vi "Periodic Tasks.vi"(8 "error in":errorcluster) -> ()   [LabVIEW 2013]
doc: "This VI runs in parallel to other tasks. It can contain as many user-defined periodic loops as you need. These can carry out PID or other sorts of timed response."
uses:
  <vilib>/Rock Robotics/SystemInterfaces/Utilities/FPGA_UtilitiesLED Source.ctl
  <vilib>/Rock Robotics/SystemInterfaces/Utilities/FPGA_UtilitiesLED State.ctl
  Robot Global Data.vi
  <vilib>/Rock Robotics/WPI/RobotDrive/WPI_RobotDriveArcadeDrive_Standard(NoSaturation).vi
panel:
  out "Rear Motor Run?":bool
  out "Front LEFT Motor Output  2":dbl
  out "Rear RIGHT Motor Output 2":dbl
  out "Front Left Net Closed?":bool
  out "Front Left Net Open?":bool
  out "Rear Right Net Closed?":bool
  out "Rear Right Net Open?":bool
  out "Front LEFT Motor Output":dbl
  out "Rear RIGHT Motor Output":dbl
  out "axis 4":dbl
  out "axis 3 (throttle)":dbl
  out "Ball Motor Output":dbl
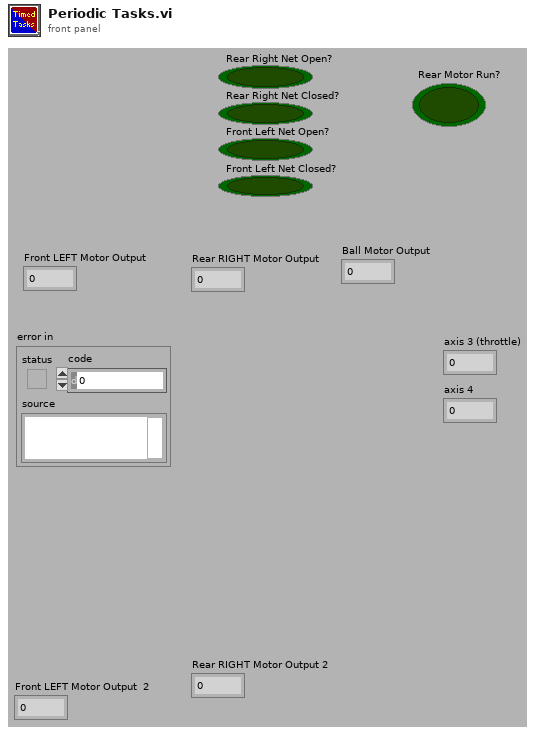
[diagram p1: front panel]
types:
  T1 = typedef "WPI_DigitalInputDevRef.ctl" = cluster{"DevStatus":errorcluster, "DIO Channel":T2, "Digital Module":T3}
  T2 = typedef "FPGA_DIOChannel.ctl" = enum8{"DIO 1", "DIO 2", "DIO 3", "DIO 4", "DIO 5", "DIO 6", "DIO 7", "DIO 8", "DIO 9", "DIO 10", "DIO 11", "DIO 12", "DIO 13", "DIO 14", "Invalid"}
  T3 = typedef "FPGA_TypedefDigitalModule.ctl" = enum16{"Digital Module 1", "Digital Module 2"}
  T4 = typedef "WPI_MotorControlDeviceRef.ctl" = cluster{"DeviceStatus":errorcluster, "Type":enum16{"PWM", "CAN"}, "PWM":cluster{"Digital Module":T3, "PWM Channel":T5, "DeadBand":T6}, "CAN":cluster{"Device Number":u8, "Control Mode":T7, "Semaphore":T8, "Max Vout":dbl}, "Invert":bool, "TransformRef":T9, "InvTransformRef":T9}
  T5 = typedef "FPGA_DIOPWMChannel.ctl" = enum8{"PWM 1", "PWM 2", "PWM 3", "PWM 4", "PWM 5", "PWM 6", "PWM 7", "PWM 8", "PWM 9", "PWM 10", "Invalid"}
  T6 = typedef "WPI_PWMDeadband.ctl" = cluster{"Name":string, "maxPositivePwm":i32, "minPositivePwm":i32, "centerPwm":i32, "maxNegativePwm":i32, "minNegativePwm":i32, "angularRange":u16}
  T7 = typedef "WPI_CANJaguar_ControlMode.ctl" = enum8{"Percent VBus", "Current", "Speed", "Position", "Voltage"}
  T8 = typedef "Semaphore RefNum" = refnum<k1>
  T9 = typedef "WPI_PWMTransform_ConPane.ctl" = refnum<vi>
  T10 = typedef "WPI_JoystickDevRef.ctl" = cluster{"Device":T11}
  T11 = typedef "WPI_JoystickDeviceEnum.ctl" = enum16{"USB 1", "USB 2", "USB 3", "USB 4", "Kinect 1", "Kinect 2"}
  T12 = typedef "WPI_RobotDriveDevRef.ctl" = cluster{"DevStatus":errorcluster, "Motors[]":T4[], "Square Inputs":bool, "Max Output":dbl, "Isochronous":bool}
  T13 = typedef "WPI_GyroDevRef.ctl" = cluster{"DevStatus":errorcluster, "Analog Module":T14, "Analog Channel":T15, "Offset":dbl, "Gain (VoltsPerDegree/Second)":dbl}
  T14 = typedef "FPGA_TypedefAnalogModule.ctl" = enum16{"Analog Module 1", "Analog Module 2"}
  T15 = typedef "FPGA_AIChannel.ctl" = enum8{"AI 1", "AI 2", "AI 3", "AI 4", "AI 5", "AI 6", "AI 7", "AI 8", "Invalid"}
  T16 = typedef "WPI_AnalogChannelDevRef.ctl" = cluster{"DevStatus":errorcluster, "Analog Module":T14, "Analog Channel":T15}
  T17 = typedef "FPGA_UtilitiesLED State.ctl" = enum16{"Off", "On", "Toggle"}
  T18 = typedef "FPGA_UtilitiesLED Source.ctl" = enum16{"User LED", "FPGA LED"}
  T19 = cluster{"axis 1 (x)":dbl, "axis 2 (y)":dbl, "axis 3 (throttle)":dbl, "axis 4":dbl, "axis 5":dbl, "axis 6":dbl}
  T20 = typedef "WPI_JoystickButtonState.ctl" = cluster{"Button 1":bool, "Button 2":bool, "Button 3":bool, "Button 4":bool, "Button 5":bool, "Button 6":bool, "Button 7":bool, "Button 8":bool, "Button 9":bool, "Button 10":bool, "Button 11":bool, "Button 12":bool}
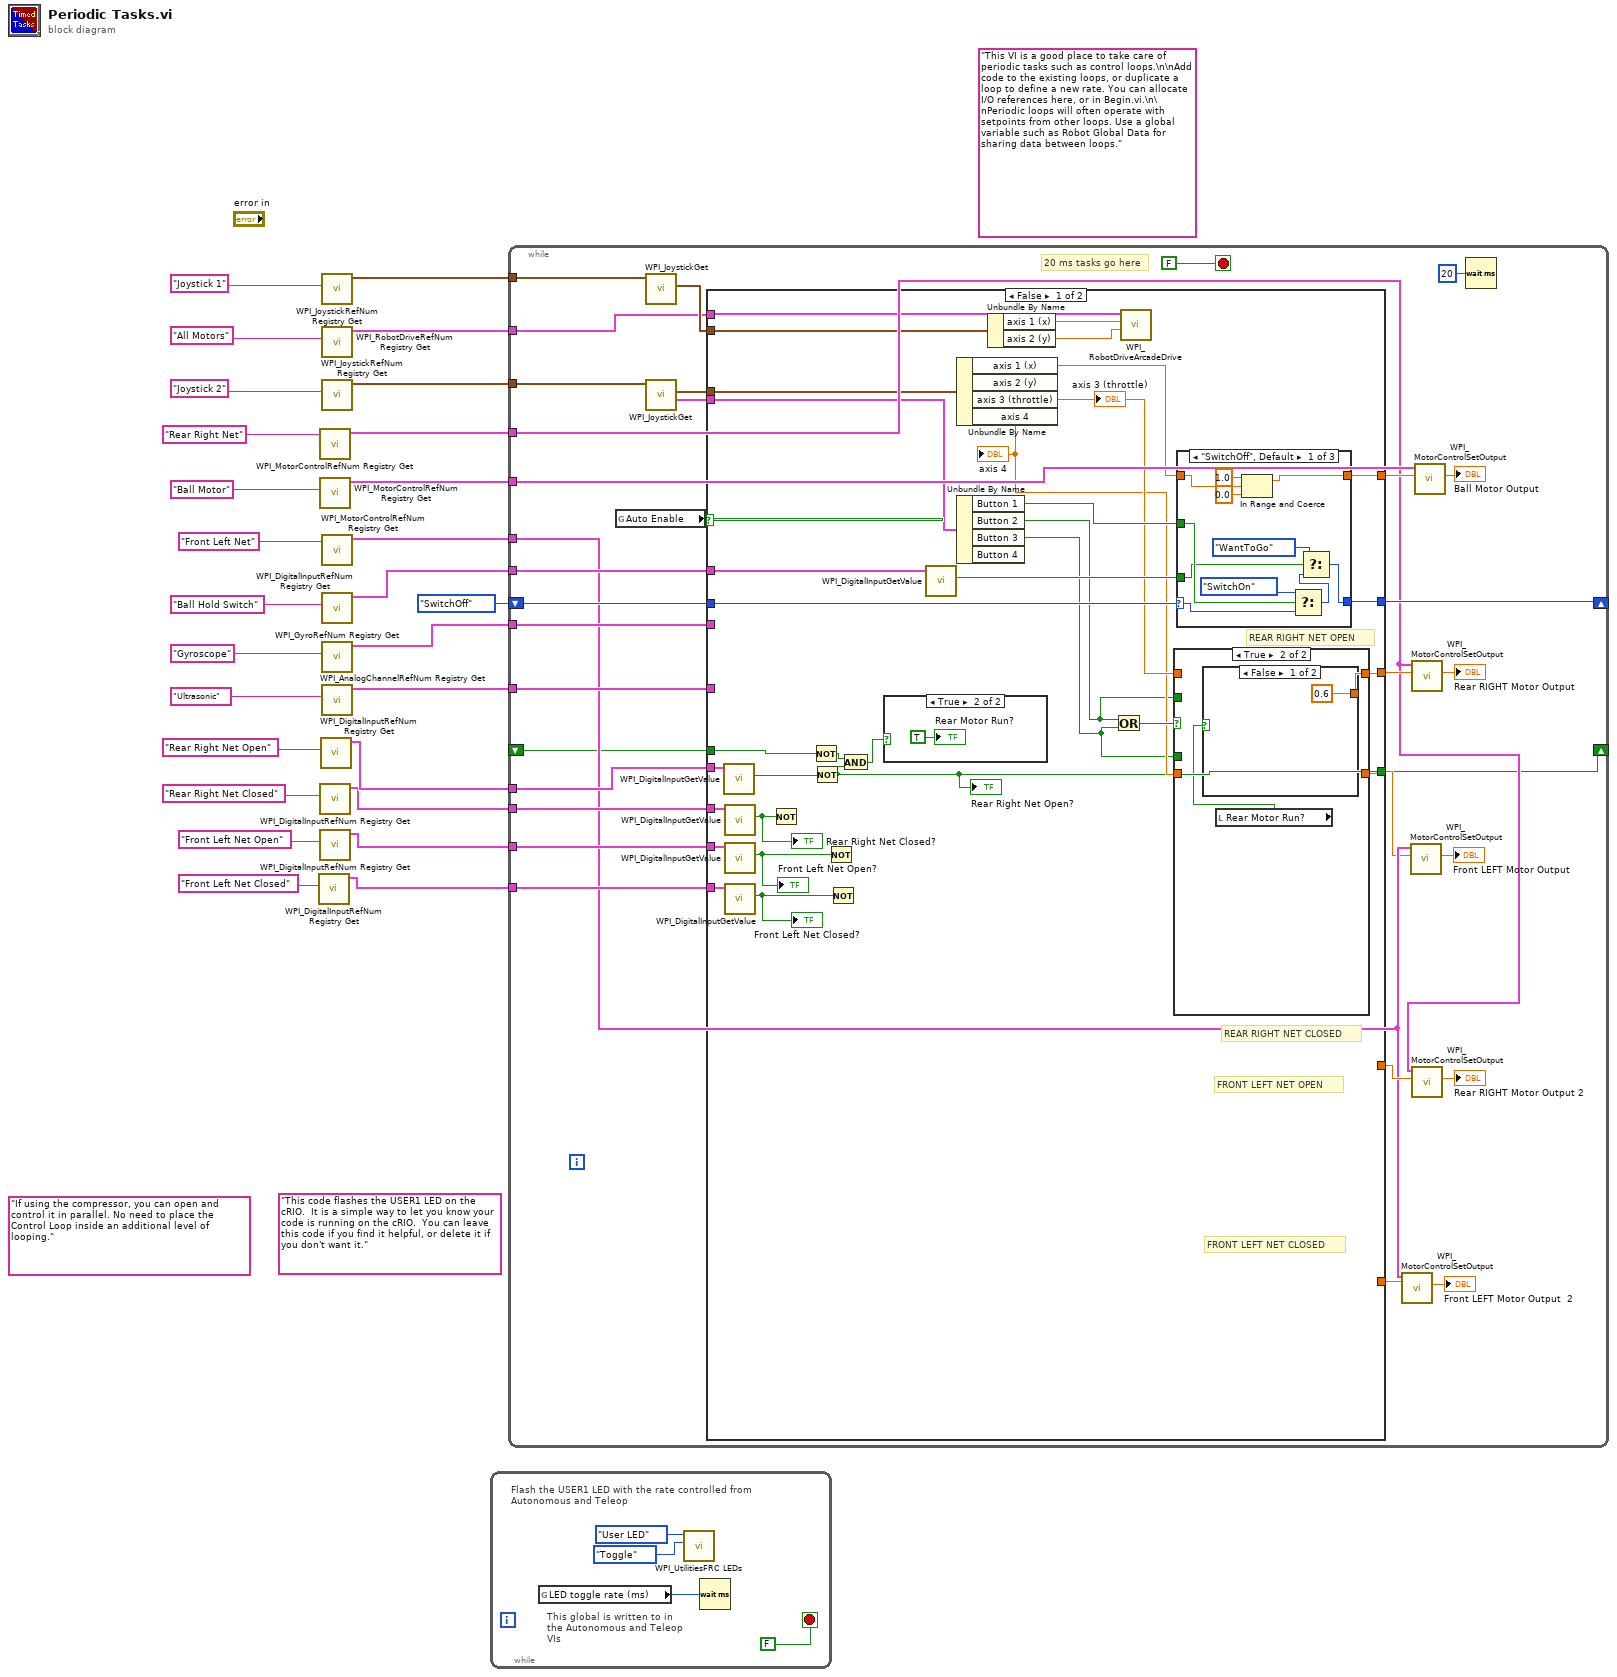
[diagram p0: block diagram]
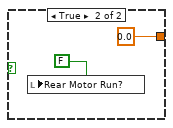
[diagram p4: hidden frame]
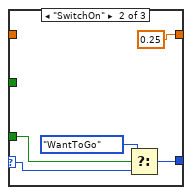
[diagram p5: hidden frame]
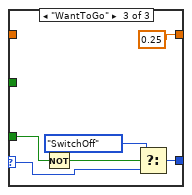
[diagram p6: hidden frame]
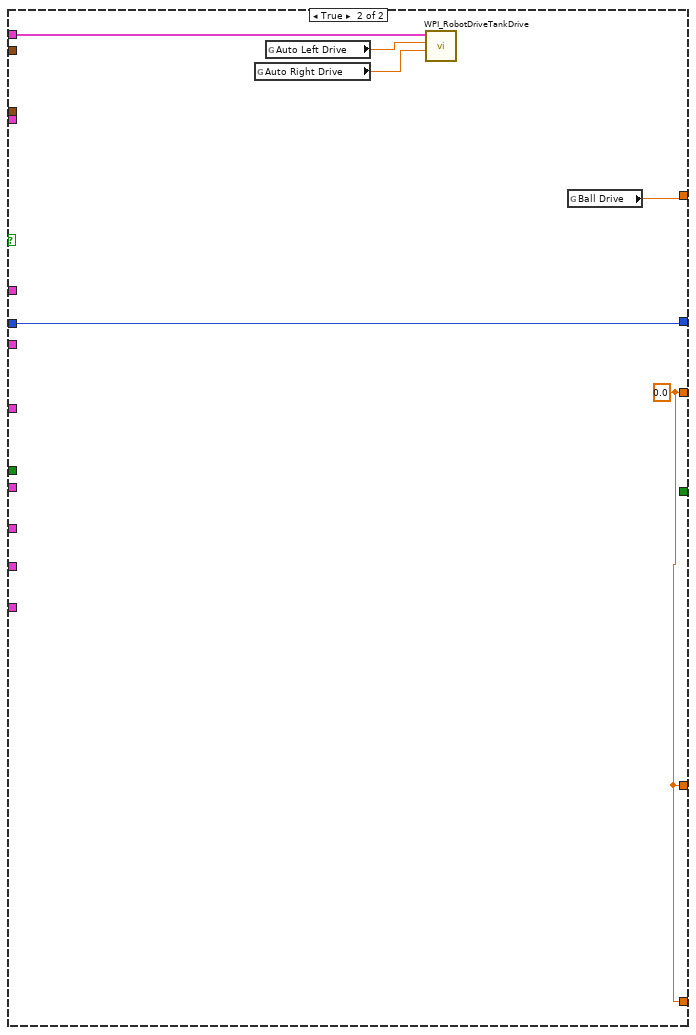
[diagram p7: hidden frame]
diagram:
  (unwired) "If using the compressor, you can open and control it in parallel. No need to place the Control Loop inside an additional level of looping."
  (unwired) "This code flashes the USER1 LED on the cRIO.  It is a simple way to let you know your code is running on the cRIO.  You can leave this code if you find it helpful, or delete it if you don't want it."
  (unwired) "This VI is a good place to take care of periodic tasks such as control loops.\n\nAdd code to the existing loops, or duplicate a loop to define a new rate. You can allocate I/O references here, or in Begin.vi.\n\nPeriodic loops will often operate with setpoints from other loops. Use a global variable such as Robot Global Data for sharing data between loops."
  n1 = call <vilib>:"WPI_DigitalInputRefNum Registry Get.vi"("refnum name"="Front Left Net Closed") -> ("DigitalInputDevRef"=w1:T1)  [unwired: 9 in, 1 out]
  n2 = call <vilib>:"WPI_MotorControlRefNum Registry Get.vi"("refnum name"="Rear Right Net") -> ("MotorControlDevRef"=w9:T4)  [unwired: 9 in, 1 out]
  n3 = call <vilib>:"WPI_MotorControlRefNum Registry Get.vi"("refnum name"="Ball Motor") -> ("MotorControlDevRef"=w11:T4)  [unwired: 9 in, 1 out]
  n4 = call <vilib>:"WPI_DigitalInputRefNum Registry Get.vi"("refnum name"="Rear Right Net Closed") -> ("DigitalInputDevRef"=w3:T1)  [unwired: 9 in, 1 out]
  n5 = call <vilib>:"WPI_DigitalInputRefNum Registry Get.vi"("refnum name"="Front Left Net Open") -> ("DigitalInputDevRef"=w2:T1)  [unwired: 9 in, 1 out]
  n6 = call <vilib>:"WPI_DigitalInputRefNum Registry Get.vi"("refnum name"="Rear Right Net Open") -> ("DigitalInputDevRef"=w4:T1)  [unwired: 9 in, 1 out]
  n7 = call <vilib>:"WPI_JoystickRefNum Registry Get.vi"("refnum name"="Joystick 1") -> ("JoystickDevRef"=w14:T10)  [unwired: 1 in, 9 out]
  n8 = call <vilib>:"WPI_RobotDriveRefNum Registry Get.vi"("refnum name"="All Motors") -> ("RobotDriveDevRef"=w13:T12)  [unwired: 1 in, 9 out]
  n9 = call <vilib>:"WPI_JoystickRefNum Registry Get.vi"("refnum name"="Joystick 2") -> ("JoystickDevRef"=w12:T10)  [unwired: 1 in, 9 out]
  n10 = call <vilib>:"WPI_MotorControlRefNum Registry Get.vi"("refnum name"="Front Left Net") -> ("MotorControlDevRef"=w10:T4)  [unwired: 9 in, 1 out]
  n11 = call <vilib>:"WPI_DigitalInputRefNum Registry Get.vi"("refnum name"="Ball Hold Switch") -> ("DigitalInputDevRef"=w21:T1)  [unwired: 9 in, 1 out]
  n12 = call <vilib>:"WPI_GyroRefNum Registry Get.vi"("refnum name"="Gyroscope") -> ("GyroDevRef"=w19:T13)  [unwired: 9 in, 1 out]
  n13 = call <vilib>:"WPI_AnalogChannelRefNum Registry Get.vi"("refnum name"="Ultrasonic") -> ("AIDeviceRef"=w17:T16)  [unwired: 9 in, 1 out]
  n14 = while {
    stop <- FALSE stop-if-true
    # "This global is written to in the Autonomous and Teleop VIs"
    # "Flash the USER1 LED with the rate controlled from Autonomous and Teleop"
    n15 = global read "Robot Global Data.vi" "LED toggle rate (ms)"() -> (w28:u32)
    n16 = call <vilib>:"WPI_UtilitiesFRC LEDs.vi"("State"=FPGA_UtilitiesLED_State."Toggle", "LED Type"=FPGA_UtilitiesLED_Source."User LED") -> ()  [unwired: 1 in, 9 out]
    n17 = Wait (ms)(milliseconds to wait=w28) -> ()  [unwired: 1 out]
  }
  n18 = while {
    shift-right: [w57] -> _
    shift-left: enum16{"SwitchOff", "SwitchOn", "WantToGo"}."SwitchOff" -> [w59]
    tunnel: w21 -> [w55]
    tunnel: w19 -> [w53]
    tunnel: w17 -> [w52]
    tunnel: w14 -> [w51]
    tunnel: w13 -> [w50]
    tunnel: w12 -> [w49]
    tunnel: w11 -> [w48]
    tunnel: w10 -> [w35]
    tunnel: w9 -> [w39]
    tunnel: w4 -> [w45]
    tunnel: w3 -> [w44]
    tunnel: w2 -> [w43]
    tunnel: w1 -> [w42]
    shift-right: [w33] -> _
    shift-left: _ -> [w32]
    stop <- FALSE stop-if-true
    # "20 ms tasks go here"
    n19 = global read "Robot Global Data.vi" "Auto Enable"() -> (w61:bool)
    n20 = call <vilib>:"WPI_JoystickGet.vi"("JoystickDevRef"=w51) -> ("Axes"=w62:T19)  [unwired: 4 in, 2 out]
    n21 = call <vilib>:"WPI_JoystickGet.vi"("JoystickDevRef"=w49) -> ("Buttons"=w54:T20, "Axes"=w60:T19)  [unwired: 4 in, 1 out]
    n22 = case shown="False" w61 {
      tunnel: w62 -> [w96 _]
      tunnel: w50 -> [w95 w132]
      tunnel: w60 -> [w86 _]
      tunnel: w59 -> [w92 w129]
      tunnel: [w91 w128] -> w58
      tunnel: [w90 w129] -> w57
      tunnel: w55 -> [w88 _]
      tunnel: w54 -> [w87 _]
      tunnel: w53 -> [_ _]
      tunnel: w52 -> [_ _]
      tunnel: w45 -> [w83 _]
      tunnel: w44 -> [w82 _]
      tunnel: w43 -> [w81 _]
      tunnel: w42 -> [w80 _]
      tunnel: [w74 w127] -> w41
      tunnel: [_ w127] -> w38
      tunnel: [_ w127] -> w36
      tunnel: [w71 _] -> w34
      tunnel: [w65 _] -> w33
      tunnel: w32 -> [w68 _]
      frame False {
        # "FRONT LEFT NET CLOSED"
        # "REAR RIGHT NET CLOSED"
        # "FRONT LEFT NET OPEN"
        # "REAR RIGHT NET OPEN"
        n23 = call <vilib>:"WPI_DigitalInputGetValue.vi"("DigitalInputDevRef"=w83) -> ("Value"=w79:bool)  [unwired: 8 in, 2 out]
        n24 = call <vilib>:"WPI_DigitalInputGetValue.vi"("DigitalInputDevRef"=w82) -> ("Value"=w77:bool)  [unwired: 8 in, 2 out]
        "Rear Right Net Closed?" <- w77
        n25 = call <vilib>:"WPI_DigitalInputGetValue.vi"("DigitalInputDevRef"=w81) -> ("Value"=w78:bool)  [unwired: 8 in, 2 out]
        "Front Left Net Open?" <- w78
        n26 = call <vilib>:"WPI_DigitalInputGetValue.vi"("DigitalInputDevRef"=w80) -> ("Value"=w76:bool)  [unwired: 8 in, 2 out]
        "Front Left Net Closed?" <- w76
        n27 = Not(x=w77) -> ()  [unwired: 1 out]
        n28 = Not(x=w68) -> (.not. x?=w67:bool)
        n29 = Not(x=w79) -> (.not. x?=w65:bool)
        "Rear Right Net Open?" <- w65
        n30 = Not(x=w78) -> ()  [unwired: 1 out]
        n31 = Not(x=w76) -> ()  [unwired: 1 out]
        n32 = And(x=w67, y=w65) -> (x .and. y?=w66:bool)
        n33 = case shown="True" w66 {
          frame False {
          }
          frame True {
            "Rear Motor Run?" <- TRUE ("Rear Right Switch State")
          }
        }
        n34 = call <vilib>:"WPI_DigitalInputGetValue.vi"("DigitalInputDevRef"=w88) -> ("Value"=w89:bool)  [unwired: 8 in, 2 out]
        n35 = Unbundle By Name(w86) -> ("axis 1 (x)"=w84:dbl, "axis 3 (throttle)"=w75:dbl, "axis 4"=w72:dbl)  [unwired: 1 out]
        "axis 3 (throttle)" <- w75
        "axis 4" <- w72
        n36 = Unbundle By Name(w87) -> ("Button 1"=w85:bool, "Button 2"=w70:bool, "Button 3"=w69:bool)  [unwired: 1 out]
        n37 = Unbundle By Name(w96) -> ("axis 1 (x)"=w94:dbl, "axis 2 (y)"=w93:dbl)
        n38 = Or(x=w70, y=w69) -> (x .or. y?=w73:bool)
        n39 = call-poly <vilib>:"WPI_RobotDriveArcadeDrive.vi"("Y axis value"=w93, "X axis value"=w94, "RobotDriveDevRef"=w95) -> ()  [unwired: 6 in, 3 out]
        n40 = case shown="True" w73 {
          tunnel: w75 -> [w99 _]
          tunnel: [w99 w100] -> w74
          tunnel: w72 -> [w98 _]
          tunnel: [w98 _] -> w71
          tunnel: w70 -> [_ _]
          tunnel: w69 -> [_ _]
          frame False {
          }
          frame True {
            n41 = local read "Rear Motor Run?"() -> (w101:bool)
            n42 = case shown="False" w101 {
              tunnel: [0.6 ("lower limit") 0.0 ("lower limit")] -> w100
              frame False {
              }
              frame True {
                n43 = local write "Rear Motor Run?"(FALSE ("Rear Right Switch State")) -> ()
              }
            }
          }
        }
        n44 = case shown="\"SwitchOff\", Default" w92 {
          selector: w92 -> [w115 w119 w122]
          tunnel: [w105 0.25 ("Output") 0.25 ("Output")] -> w91
          tunnel: w89 -> [w109 w117 w121]
          tunnel: [w110 w116 w123] -> w90
          tunnel: w85 -> [w113 _ _]
          tunnel: w84 -> [w108 _ _]
          frame "SwitchOff", Default {
            n45 = In Range and Coerce(upper limit=1.0, x=w108, lower limit=0.0) -> (coerced(x)=w105:dbl)  [unwired: 1 out]
            n46 = Select(t=enum16{"SwitchOff", "SwitchOn", "WantToGo"}."SwitchOn", s=w113, f=w115) -> (s? t:f=w111:enum16{"SwitchOff", "SwitchOn", "WantToGo"})
            n47 = Select(t=enum16{"SwitchOff", "SwitchOn", "WantToGo"}."WantToGo", s=w109, f=w111) -> (s? t:f=w110:enum16{"SwitchOff", "SwitchOn", "WantToGo"})
          }
          frame "SwitchOn" {
            n48 = Select(t=enum16{"SwitchOff", "SwitchOn", "WantToGo"}."WantToGo", s=w117, f=w119) -> (s? t:f=w116:enum16{"SwitchOff", "SwitchOn", "WantToGo"})
          }
          frame "WantToGo" {
            n49 = Not(x=w121) -> (.not. x?=w125:bool)
            n50 = Select(t=enum16{"SwitchOff", "SwitchOn", "WantToGo"}."SwitchOff", s=w125, f=w122) -> (s? t:f=w123:enum16{"SwitchOff", "SwitchOn", "WantToGo"})
          }
        }
      }
      frame True {
        w127 = 0.0 ("Output")
        n51 = global read "Robot Global Data.vi" "Auto Right Drive"() -> (w130:dbl)
        n52 = global read "Robot Global Data.vi" "Auto Left Drive"() -> (w131:dbl)
        n53 = call <vilib>:"WPI_RobotDriveTankDrive.vi"("Right axis value"=w130, "Left axis value"=w131, "RobotDriveDevRef"=w132) -> ()  [unwired: 6 in, 3 out]
        n54 = global read "Robot Global Data.vi" "Ball Drive"() -> (w128:dbl)
      }
    }
    n55 = call <vilib>:"WPI_MotorControlSetOutput.vi"("Output"=w36, "MotorControlDevRef"=w35) -> ("Motor Output"=→"Front LEFT Motor Output  2":dbl)  [unwired: 7 in, 2 out]
    n56 = call <vilib>:"WPI_MotorControlSetOutput.vi"("Output"=w34, "MotorControlDevRef"=w35) -> ("Motor Output"=→"Front LEFT Motor Output":dbl)  [unwired: 7 in, 2 out]
    n57 = call <vilib>:"WPI_MotorControlSetOutput.vi"("Output"=w41, "MotorControlDevRef"=w39) -> ("Motor Output"=→"Rear RIGHT Motor Output":dbl)  [unwired: 7 in, 2 out]
    n58 = call <vilib>:"WPI_MotorControlSetOutput.vi"("Output"=w38, "MotorControlDevRef"=w39) -> ("Motor Output"=→"Rear RIGHT Motor Output 2":dbl)  [unwired: 7 in, 2 out]
    n59 = call <vilib>:"WPI_MotorControlSetOutput.vi"("Output"=w58, "MotorControlDevRef"=w48) -> ("Motor Output"=→"Ball Motor Output":dbl)  [unwired: 7 in, 2 out]
    n60 = Wait (ms)(milliseconds to wait=u32 20) -> ()  [unwired: 1 out]
  }
